vi "Get Index.vi"(8 "error in (no error)":errorcluster, 11 "Vector Parent in":refnum<class "Vector Parent.lvclass">) -> (0 "error out":errorcluster, 2 "Index":i32, 3 "Vector Parent out":refnum<class "Vector Parent.lvclass">)   [LabVIEW 2019, in "Vector Parent.lvclass"]
uses:
  Vector Parent.lvclass
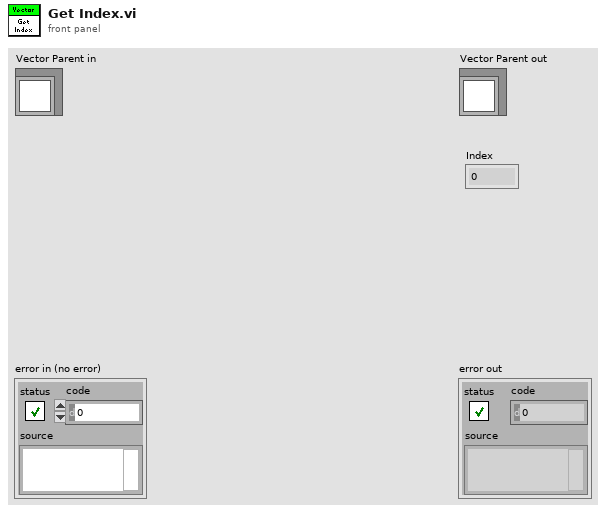
[diagram p1: front panel]
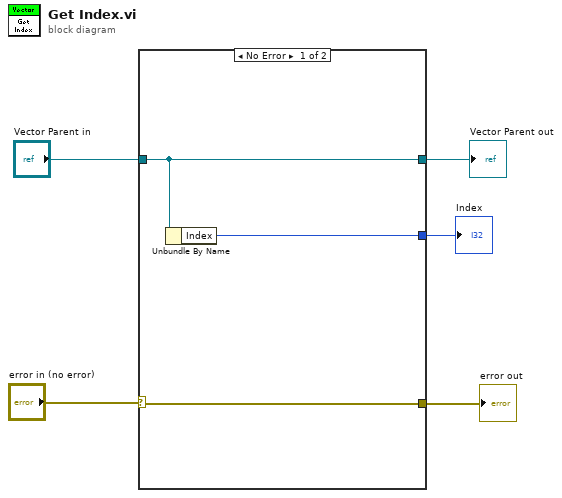
[diagram p0: block diagram]
diagram:
  n1 = case shown="No Error" "error in (no error)" {
    selector: "error in (no error)" -> [w8 w10]
    tunnel: "Vector Parent in" -> [w7 w9]
    tunnel: [w7 w9] -> w3
    tunnel: [w8 w10] -> w2
    tunnel: [w6 _] -> w1
    frame No Error {
      n2 = Unbundle By Name(w7) -> ("Index"=w6:i32)
    }
    frame Error {
    }
  }
  "error out" <- w2
  "Vector Parent out" <- w3
  "Index" <- w1
